vi "Handle Results.vi"(8 "error in (no error)":errorcluster, 11 "Results":T1[](array[typedef])) -> (0 "error out":errorcluster, 2 "Result":bool)   [LabVIEW 2020, in "SoL Inspector.lvlib"]
uses:
  SoL Inspector.lvlib
  Inspection Result.ctl
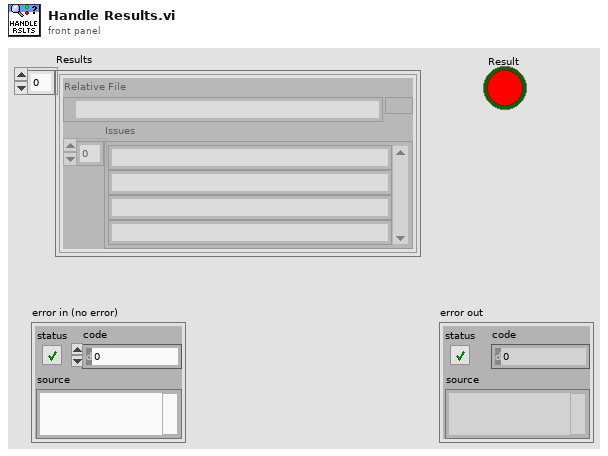
[diagram p1: front panel]
types:
  T1 = typedef "SoL Inspector.lvlib/Inspection Result.ctl" = cluster{"Relative File":path, "Issues":string[]}
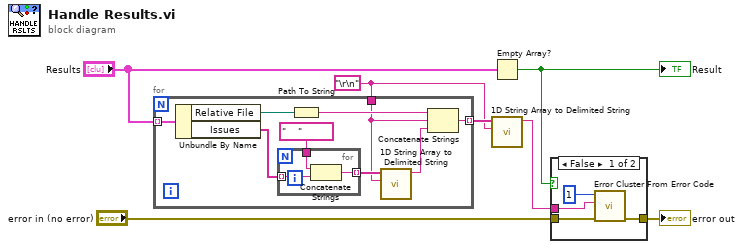
[diagram p0: block diagram]
diagram:
  w4 = "\r\n"
  n1 = for {
    tunnel: "Results" -> [w16] mode=indexing
    tunnel: [w10] -> w5 mode=indexing
    tunnel: w4 -> [w8]
    n2 = Unbundle By Name(w16) -> ("Relative File"=w12:path, "Issues"=w15:string[])
    n3 = for {
      tunnel: w15 -> [w19] mode=indexing
      tunnel: "    " -> [w18]
      tunnel: [w17] -> w13 mode=indexing
      n4 = Concatenate Strings(w18, w19) -> (w17:string)
    }
    n5 = Path To String(path=w12) -> (string=w11:string)
    n6 = call <vilib>:"1D String Array to Delimited String.vi"("delimiter"=w8, "string array"=w13) -> ("delimited string"=w9:string)  [unwired: 9 in]
    n7 = Concatenate Strings(w11, w8, w9) -> (w10:string)
  }
  n8 = Empty Array?(array="Results") -> (empty?=w7:bool)
  "Result" <- w7
  n9 = call <vilib>:"1D String Array to Delimited String.vi"("delimiter"=w4, "string array"=w5) -> ("delimited string"=w3:string)  [unwired: 9 in]
  n10 = case shown="False" w7 {
    tunnel: "error in (no error)" -> [w23 w24]
    tunnel: [w22 w24] -> w1
    tunnel: w3 -> [w20 _]
    frame False {
      n11 = call <vilib>:"Error Cluster From Error Code.vi"("error in (no error)"=w23, "error message (\"\")"=w20, "error code (0)"=1) -> ("error out"=w22:errorcluster)  [unwired: 6 in]
    }
    frame True {
    }
  }
  "error out" <- w1
